vi "Get Firmware Version.vi"(3 "error in":errorcluster) -> (0 "error out":errorcluster, 1 "pnFwVersion":i32, 2 "return value":i32)   [LabVIEW 2015]
doc: "Description:\nThis test will return the version number of the firmware running in the Cypress.\nDetail:\nint MEScope_GetFirmwareVer (\nint * pnFwVersion\n);\nParameters:\nint * pnFwVersion- Pointer to a integer buffer, filled with the version number data.\n\nReturn Values:\nA returned value of 0 indicates success, with the appropriate strings in the buffer. Otherwise, treat the returned value as an error code.\nRemarks:"
uses:
  ScannerDiagDLL.dll
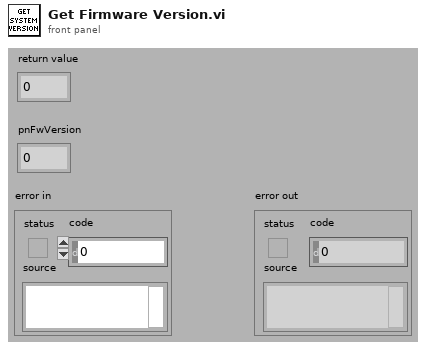
[diagram p1: front panel]
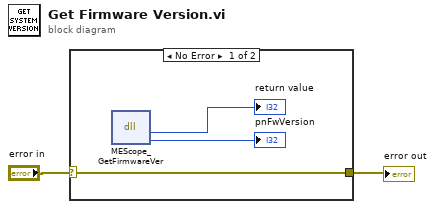
[diagram p0: block diagram]
diagram:
  n1 = case shown="No Error" "error in" {
    selector: "error in" -> [w3 w6]
    tunnel: [w3 w6] -> w1
    frame No Error {
      n2 = dll-call lib="C:/ModisEdge/Scope/Test Sequence/Code Modules/DLL/ScannerDiagDLL.dll" fn="MEScope_GetFirmwareVer"() -> ("return type"=→"return value":i32, "pnFwVersion"=→"pnFwVersion":i32)  [unwired: 4 in, 2 out]
    }
    frame Error {
    }
  }
  "error out" <- w1
